vi "PP.PNG.Encode.vi"(4 "Data Owerwrite (T)":bool=TRUE, 6 "Encode Format":T1=enum."Normal Flatten", 7 "Data":variant, 8 "error in":errorcluster, 10 "Destination PNG (default: empty)":path, 11 "PNG In":path) -> (0 "error out":errorcluster)   [LabVIEW 2020, in "PixPack.lvlib"]
doc: "This LabVIEW VI enables embedding custom data into PNG image files by appending the data to the end of the file’s byte stream. The process does not modify the visual content of the image, ensuring it remains viewable in any standard image viewer while carrying additional hidden information.\n\n<b>Usage</b>\n\n1. Specify the path to the original PNG file.\n\n2. Define the output path for the new PNG file.\n\n3. Provide any data to the Data input – this will be appended to the image file.\n\n4. (Optional) Enable XML output to save the data in an XML file instead.\n\n5. <b>If the new file input is empty, the source file will be overwritten.</b>\n\n<b>Possible Use Cases</b>\n\n - Data + Image packaging: Attach measurement data or analysis results directly to the corresponding image.\n\n - Metadata storage: Add experiment details, configuration parameters, or version info to image files.\n\n - Lightweight data transport: Send both visual and numerical information in a single portable PNG file.\n\n - Hidden annotations: Store notes or instructions inside an image without affecting its appearance."
uses:
  PixPack.lvlib
  private/User.Encode.Format.ctl
  private/Encode.Format.ctl
  <vilib>/Utility/error.llb/Error Cluster From Error Code.vi
  <vilib>/ErrorRing/Error Ring.xnode
panel:
  # "IN"
  # "OUT"
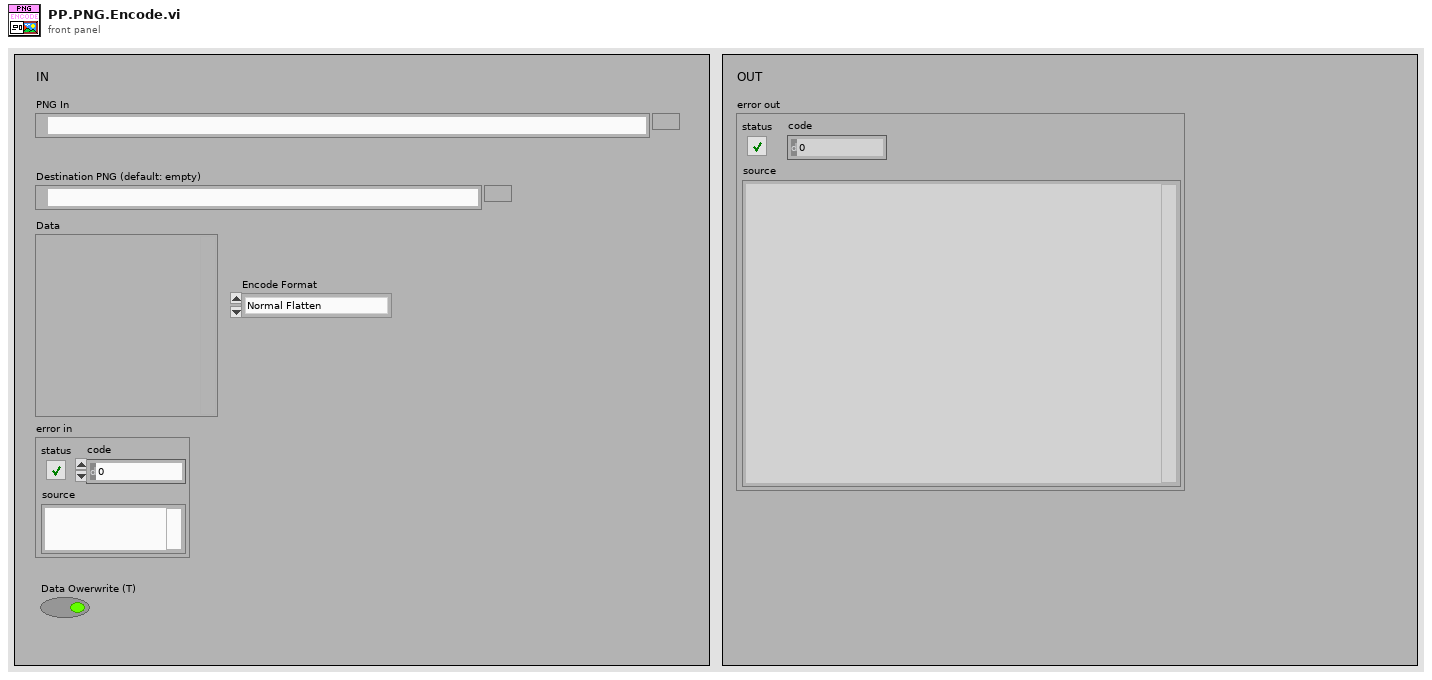
[diagram p1: front panel]
types:
  T1 = typedef "PixPack.lvlib/User.Encode.Format.ctl" = enum16{"XML Encode", "Normal Flatten", "External File"}
  T2 = typedef "PixPack.lvlib/Encode.Format.ctl" = enum16{"PIX_NOR_FLAT", "PIX_XFLAT", "PIX_EXT_FILE", "PIX_NOT_ENCODED"}
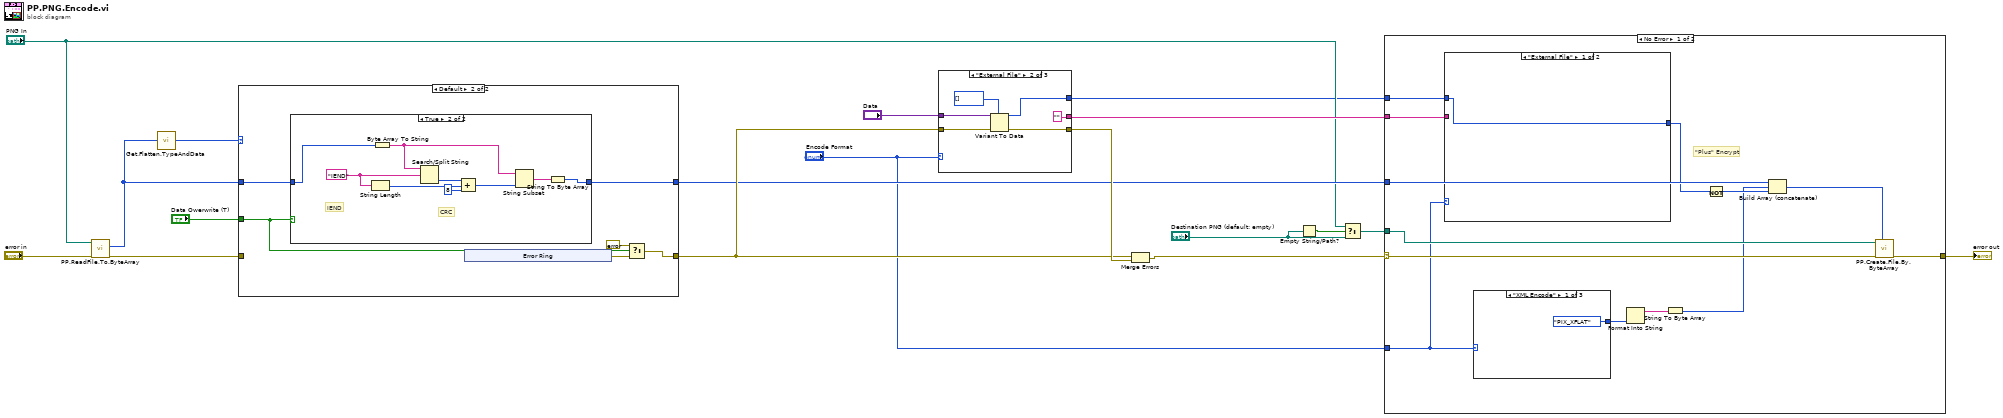
[diagram p0: block diagram]
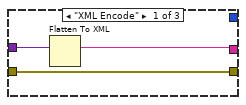
[diagram p4: hidden frame]
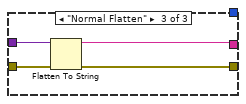
[diagram p5: hidden frame]
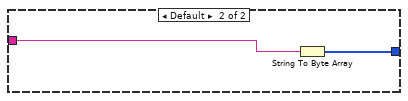
[diagram p6: hidden frame]
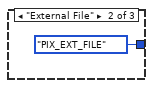
[diagram p7: hidden frame]
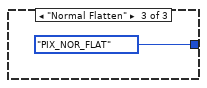
[diagram p8: hidden frame]
diagram:
  n1 = call "PP.ReadFile.To.ByteArray.vi"("error in"="error in", "file path (use dialog)"="PNG In") -> ("error out"=w3:errorcluster, "data"=w4:u8[])  [unwired: 7 in, 1 out]
  n2 = call "Get.Flatten.TypeAndData.vi"("PNG U8 Data"=w4) -> ("Flat Type"=w7:T2)  [unwired: 2 in, 2 out]
  n3 = case shown="Default" w7 {
    tunnel: w3 -> [w20 _]
    tunnel: [w20 w24] -> w10
    tunnel: "Data Owerwrite (T)" -> [_ w21]
    tunnel: w4 -> [w19 w23]
    tunnel: [w19 w22] -> w8
    frame "PIX_NOT_ENCODED" {
    }
    frame Default {
      n4 = case shown="True" w21 {
        tunnel: w23 -> [w27 w31]
        tunnel: [w27 w28] -> w22
        frame False {
        }
        frame True {
          w34 = "IEND" ("search string/char (-)")
          # "IEND"
          # "CRC"
          n5 = String Length(string=w34) -> (length=w35:i32)
          n6 = Byte Array To String(unsigned byte array=w31) -> (string=w30:string)
          n7 = Search/Split String(string=w30, search string/char (-)=w34) -> (offset of match=w32:i32)  [unwired: 1 in, 2 out]
          n8 = Compound Arithmetic op=ADD(w32, w35, 8 ("value")) -> (w33:i32)
          n9 = String Subset(string=w30, length (rest)=w33) -> (substring=w29:string)  [unwired: 1 in]
          n10 = String To Byte Array(string=w29) -> (unsigned byte array=w28:u8[])
        }
      }
      n11 = xnode "Error Ring"() -> ("error out"=w25:errorcluster)
      n12 = Select(t=errorcluster {"status"=FALSE, "code"=0, "source"=""}, s=w21, f=w25) -> (s? t:f=w24:errorcluster)
    }
  }
  n13 = case shown="\"External File\"" "Encode Format" {
    tunnel: [w42 "" ("data string") w54] -> w18
    tunnel: "Data" -> [w44 w48 w53]
    tunnel: [w43 w45 w52] -> w15
    tunnel: w10 -> [w43 w50 w51]
    tunnel: [_ w47 _] -> w1
    frame "XML Encode" {
      n14 = Flatten To XML(6:w44) -> (2:w42:string)
    }
    frame "External File" {
      n15 = Variant To Data(error in=w50, type=u8[] [] ("u8 file data"), Variant=w48) -> (data=w47:u8[], error out=w45:errorcluster)
    }
    frame "Normal Flatten" {
      n16 = Flatten To String(anything=w53, error in (no error)=w51) -> (data string=w54:string, error out=w52:errorcluster)  [unwired: 2 in, 1 out]
    }
  }
  n17 = Merge Errors(w10, w15) -> (w16:errorcluster)
  n18 = Empty String/Path?(string/path="Destination PNG (default: empty)") -> (empty?=w13:bool)
  n19 = Select(t="PNG In", s=w13, f="Destination PNG (default: empty)") -> (s? t:f=w11:path)
  n20 = case shown="No Error" w16 {
    selector: w16 -> [w62 w74]
    tunnel: w18 -> [w67 _]
    tunnel: w8 -> [w66 _]
    tunnel: [w61 w74] -> w17
    tunnel: w11 -> [w63 _]
    tunnel: "Encode Format" -> [w56 _]
    tunnel: w1 -> [w55 _]
    frame No Error {
      # "\"Plus\" Encrypt"
      n21 = case shown="\"External File\"" w56 {
        tunnel: w67 -> [_ w69]
        tunnel: [w68 w70] -> w65
        tunnel: w55 -> [w68 _]
        frame "External File" {
        }
        frame Default {
          n22 = String To Byte Array(string=w69) -> (unsigned byte array=w70:u8[])
        }
      }
      n23 = case shown="\"XML Encode\"" w56 {
        tunnel: [Encode.Format."PIX_XFLAT" ("Encode Format") Encode.Format."PIX_EXT_FILE" ("Encode Format") Encode.Format."PIX_NOR_FLAT" ("Encode Format")] -> w59
        frame "XML Encode" {
        }
        frame "External File" {
        }
        frame "Normal Flatten" {
        }
      }
      n24 = Format Into String(w59) -> (resulting string=w58:string)  [unwired: 3 in, 1 out]
      n25 = String To Byte Array(string=w58) -> (unsigned byte array=w57:u8[])
      n26 = Not(x=w65) -> (.not. x?=w64:u8[])
      n27 = Build Array (concatenate)(w66, w57, w64) -> (w60:u8[])
      n28 = call "PP.Create.File.By.ByteArray.vi"("u8 Data[]"=w60, "error in"=w62, "file path (use dialog)"=w63) -> ("error out"=w61:errorcluster)  [unwired: 7 in, 1 out]
    }
    frame Error {
    }
  }
  "error out" <- w17
